vi "DAQ Initialize.vi"(8 "error in (no error)":errorcluster caption="错误输入（无错误）") -> (0 "error out":errorcluster caption="错误输出", 1 "DAQ Tasks":T1 caption="DAQ任务", 2 "Timing Source":string caption="定时源")   [LabVIEW 2013]
uses:
  controls/DAQ Tasks.ctl
  Globals/Global - Configuration Options.vi
  <vilib>/DAQmx/create/channels.llb/DAQmx Create Virtual Channel.vi
  <vilib>/DAQmx/configure/timing.llb/DAQmx Timing.vi
  <vilib>/DAQmx/create/timing.llb/DAQmx Create Timing Source.vi
  <vilib>/DAQmx/create/timing.llb/DAQmx Create Timing Source (Control Loop From Task).vi
  <resource>/objmgr/daqmx.rc
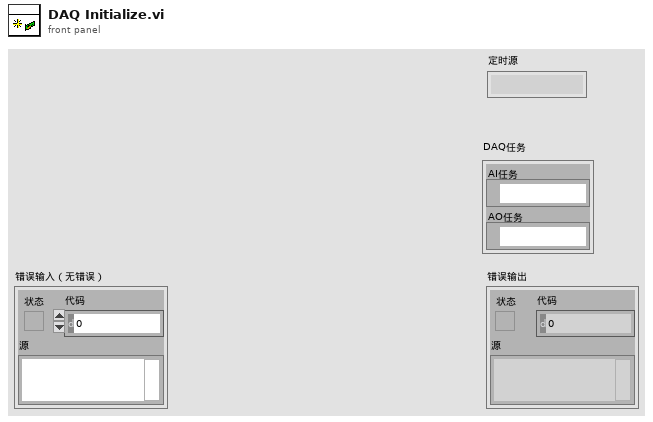
[diagram p1: front panel]
types:
  T1 = typedef "DAQ Tasks.ctl" = cluster{"AI Task":refnum<k21>, "AO Task":refnum<k21>}
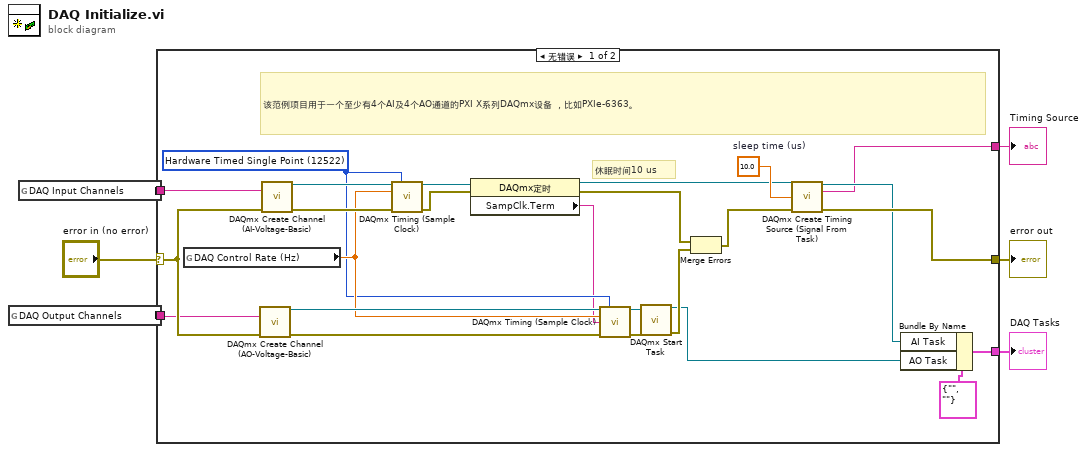
[diagram p0: block diagram]
diagram:
  n1 = global read "Global - Configuration Options.vi" "DAQ Output Channels"() -> (w1:tag)
  n2 = global read "Global - Configuration Options.vi" "DAQ Input Channels"() -> (w2:tag)
  n3 = case shown="无错误" "error in (no error)" {
    selector: "error in (no error)" -> [w14 w32]
    tunnel: [w18 w32] -> w5
    tunnel: [w30 _] -> w4
    tunnel: [w16 _] -> w3
    tunnel: w2 -> [w12 _]
    tunnel: w1 -> [w13 _]
    frame No Error {
      w15 = 10.0  # sleep time (us)
      w20 = 12522 items=["Finite Samples"=10178, "Continuous Samples"=10123, "Hardware Timed Single Point"=12522] ("sample mode")
      # "休眠时间10 us"
      # "该范例项目用于一个至少有4个AI及4个AO通道的PXI X系列DAQmx设备 ，比如PXIe-6363。"
      n4 = global read "Global - Configuration Options.vi" "DAQ Control Rate (Hz)"() -> (w21:dbl)
      n5 = call-poly <vilib>:"DAQmx Create Channel (AO-Voltage-Basic).vi"("physical channels"=w13, "error in"=w14) -> ("task out"=w24:refnum<k21>, "error out"=w25:errorcluster)  [unwired: 12 in]
      n6 = call-poly <vilib>:"DAQmx Create Channel (AI-Voltage-Basic).vi"("physical channels"=w12, "error in"=w14) -> ("task out"=w23:refnum<k21>, "error out"=w22:errorcluster)  [unwired: 12 in]
      n7 = call-poly <vilib>:"DAQmx Timing (Sample Clock).vi"("task/channels in"=w23, "sample mode"=w20, "rate"=w21, "error in"=w22) -> ("task out"=w11:refnum<k21>, "error out"=w8:errorcluster)  [unwired: 10 in]
      n8 = property class="DAQmx定时"(reference=w11, error in=w8) -> (reference out=w10:refnum<k21>, error out=w7:errorcluster, "SampClk.Term"=w9:tag)
      n9 = call-poly <vilib>:"DAQmx Timing (Sample Clock).vi"("task/channels in"=w24, "sample mode"=w20, "rate"=w21, "source"=w9, "error in"=w25) -> ("task out"=w28:refnum<k21>, "error out"=w29:errorcluster)  [unwired: 9 in]
      n10 = call <vilib>:"DAQmx Start Task.vi"("task/channels in"=w28, "error in"=w29) -> ("task out"=w19:refnum<k21>, "error out"=w26:errorcluster)  [unwired: 12 in]
      n11 = Merge Errors(w7, w26) -> (w27:errorcluster)
      n12 = call-poly "DAQmx Create Timing Source (Signal From Task).vi"("task/channels in"=w10, "sleep time (us)"=w15, "error in"=w27) -> ("task out"=w17:refnum<k21>, "timing source out"=w16:string, "error out"=w18:errorcluster)  [unwired: 10 in]
      n13 = Bundle By Name(cluster=T1 {"AI Task"="", "AO Task"=""} ("DAQ Tasks"), "AI Task"=w17, "AO Task"=w19) -> (w30:T1)
    }
    frame Error {
    }
  }
  "error out" <- w5
  "Timing Source" <- w3
  "DAQ Tasks" <- w4
